vi "Find Packed Library.vi"(8 "error in (no error)":errorcluster, 10 "packed library name":string, 11 "Component Loader in":refnum<class "Component Loader.lvclass">) -> (0 "error out":errorcluster, 2 "packed library path":path, 3 "Component Loader out":refnum<class "Component Loader.lvclass">)   [LabVIEW 2017, in "DSF Core.lvlib" / "Component Loader.lvclass"]
uses:
  Component Loader.lvclass
  Component Not Found.vi
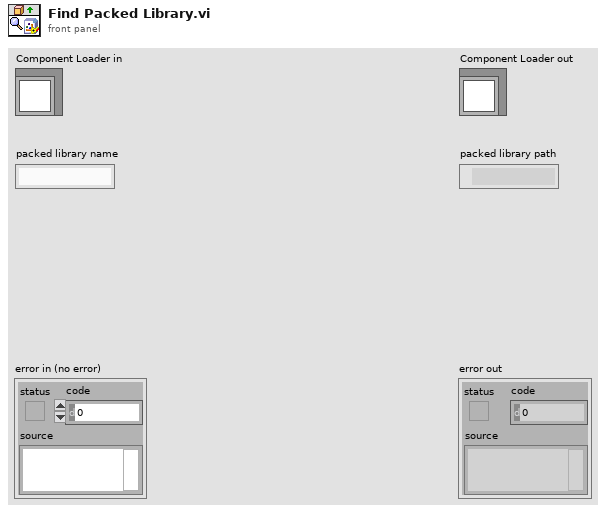
[diagram p1: front panel]
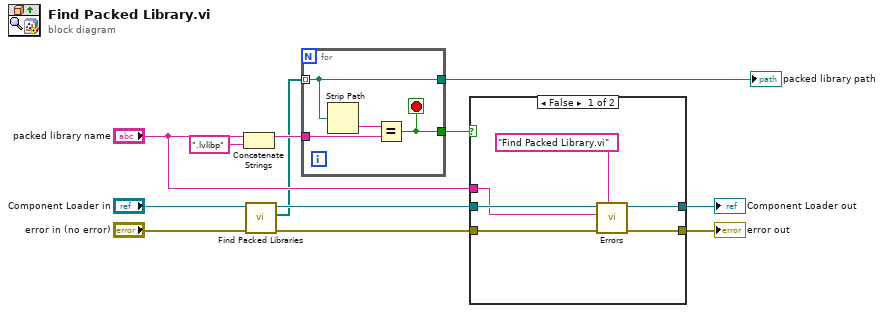
[diagram p0: block diagram]
diagram:
  n1 = Concatenate Strings("packed library name", ".lvlibp" ("string")) -> (w3:string)
  n2 = call "Find Packed Libraries.vi"("error in (no error)"="error in (no error)", "Component Loader in"="Component Loader in") -> ("error out"=w7:errorcluster, "packed library paths"=w1:path[], "Component Loader out"=w8:refnum<class "Component Loader.lvclass">)  [unwired: 7 in]
  n3 = for {
    tunnel: w1 -> [w14] mode=indexing
    tunnel: w3 -> [w15]
    tunnel: [w14] -> w10
    tunnel: [w13] -> w9
    stop <- w13 stop-if-true
    n4 = Strip Path(path=w14) -> (name=w16:string)  [unwired: 1 out]
    n5 = Equal?(x=w16, y=w15) -> (x = y?=w13:bool)
  }
  "packed library path" <- w10
  n6 = case shown="False" w9 {
    tunnel: w8 -> [w22 w24]
    tunnel: w7 -> [w21 w23]
    tunnel: [w20 w24] -> w6
    tunnel: [w19 w23] -> w5
    tunnel: "packed library name" -> [w18 _]
    frame False {
      n7 = call-poly "Errors.vi"("error source vi name"="Find Packed Library.vi", "error in (no error)"=w21, "component name"=w18, "Component Loader in"=w22) -> ("error out"=w19:errorcluster, "Component Loader out"=w20:refnum<class "Component Loader.lvclass">)  [unwired: 6 in]
    }
    frame True {
    }
  }
  "error out" <- w5
  "Component Loader out" <- w6
